vi "TEG P116x2w_Write_Manual.vi"(7 "MaxOutput":T1={"Ch1"=100.0, "Ch2"=100.0}, 8 "error in (no error)":errorcluster, 9 "RateSP":T1, 10 "NuevoSP":T1, 11 "Comunicaciones":T2={"Alicats"="ASRL6::INSTR", "Alic"=FALSE, "eValve"="ASRL6::INSTR", "eval"=FALSE, "Eurotherm"="ASRL6::INSTR", "euro"=FALSE, "Cell GAS"="ASRL6::INSTR", "cgas"=FALSE, "Cell H2S"="ASRL6::INSTR", "ch2s"=FALSE}) -> (0 "error out":errorcluster, 1 "RateSP(C/min) 2":T1, 2 "NuevoSP(C) 2":T1, 3 "MaxOutput 2":T1)   [LabVIEW 2017]
uses:
  2xP116.ctl
  REACTOR_COMUNICACIONES.ctl
  Eurotherm_2023_Module.ctl
  REACTOR_GLOBALES.vi
panel:
  out "Temp":T1
  in  "Cancel":bool
  in  "OK":bool
  out "Enable(T)":bool=TRUE
  out "VISA Promux":refnum<visa-resource-name>
  in  "Delay Time (s)":dbl=0.1
  # "Programando controladores P116"
  # "C"
  # "%"
  # "CALOR"
  # "C/min"
  # "C"
  # "%"
  # "FRIO"
  # "C/min"
  # "NOTA: La válvula de \"aire frio\" se conectará cuando \nla temperatura del reactor supere la temperatura \nNuevoSP FRIO establecida"
  # "Abril 2023 V1.0  a-sslcdms"
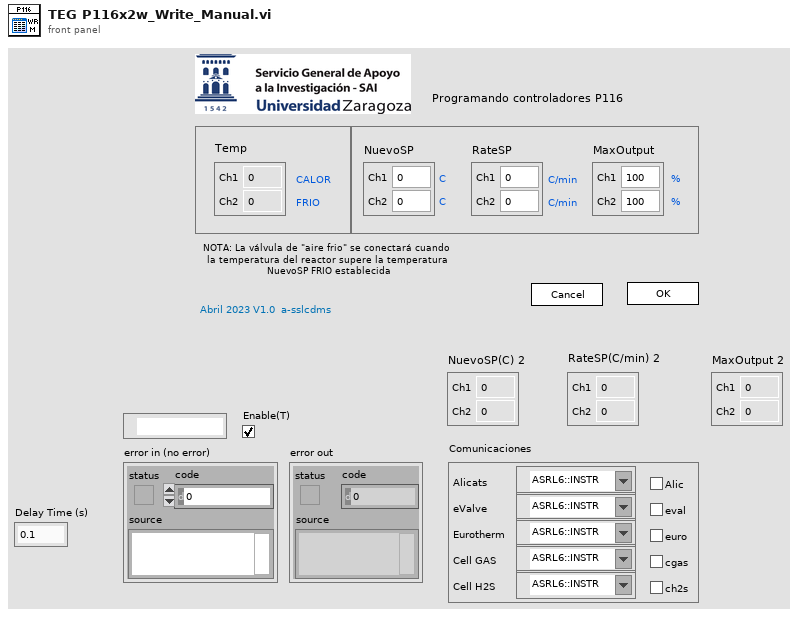
[diagram p1: front panel]
types:
  T1 = typedef "2xP116.ctl" = cluster{"Ch1":dbl, "Ch2":dbl}
  T2 = typedef "REACTOR_COMUNICACIONES.ctl" = cluster{"Alicats":refnum<visa-resource-name>, "Alic":bool, "eValve":refnum<visa-resource-name>, "eval":bool, "Eurotherm":refnum<visa-resource-name>, "euro":bool, "Cell GAS":refnum<visa-resource-name>, "cgas":bool, "Cell H2S":refnum<visa-resource-name>, "ch2s":bool}
  T3 = typedef "TEG P116x2w.ctl" = cluster{"TargetSP":T1, "WorkingSP":T1, "Temperatura":T1, "Error":bool, "Date":string, "Delay(s)":dbl, "RateSP":T1, "Potencia":T1, "Potencia max":T1}
  T4 = typedef "Eurotherm_2023_Module.ctl" = enum16{"Initialize", "Write setpoint", "Read data", "Write ramp rate", "Set constante proporcional", "Set constante integral", "Set constante diferencial", "Set ouput limit LOW", "Set ouput limit HIGH", "Shutdown"}
  T5 = enum16{"Add 1", "Add 2", "Add 3", "Add 10", "Add 11", "Add 12", "Add 13"}[]
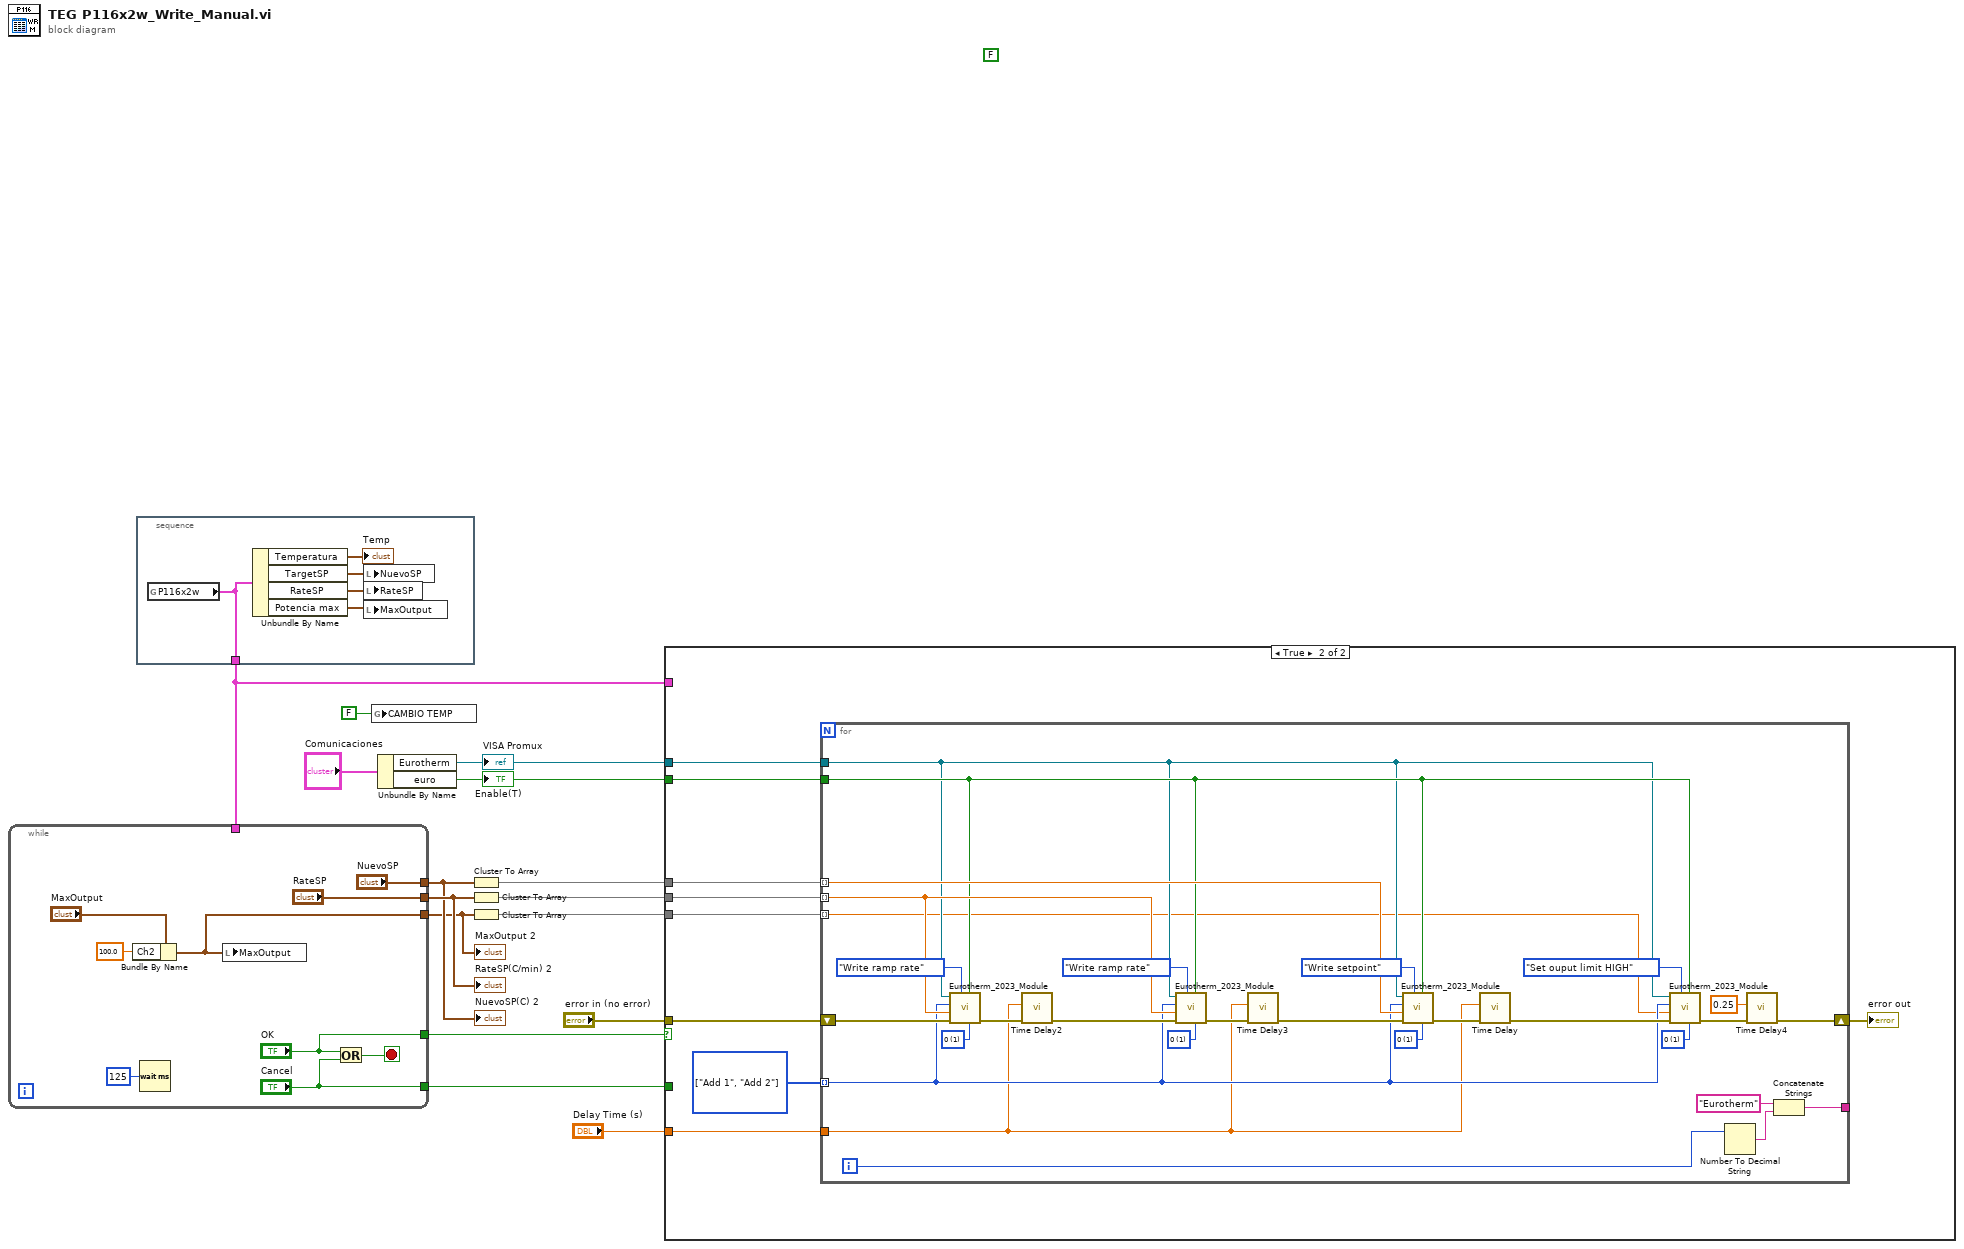
[diagram p0: block diagram]
diagram:
  (unwired) FALSE
  n1 = stacked-sequence {
    tunnel: [w18] -> w7
    frame #0 {
      n2 = global read "REACTOR_GLOBALES.vi" "P116x2w"() -> (w18:T3)
      n3 = Unbundle By Name(w18) -> ("Temperatura"=→"Temp":T1, "TargetSP"=w19:T1, "RateSP"=w17:T1, "Potencia max"=w16:T1)
      n4 = local write "NuevoSP"(w19) -> ()
      n5 = local write "RateSP"(w17) -> ()
      n6 = local write "MaxOutput"(w16) -> ()
    }
  }
  n7 = while {
    tunnel: ["Cancel"] -> w14
    tunnel: ["NuevoSP"] -> w3
    tunnel: ["RateSP"] -> w6
    tunnel: ["OK"] -> w10
    tunnel: w7 -> [_]
    tunnel: [w21] -> w2
    stop <- w24 stop-if-true
    n8 = Bundle By Name(cluster="MaxOutput", "Ch2"=100.0) -> (w21:T1)
    n9 = Wait (ms)(milliseconds to wait=u32 125) -> ()  [unwired: 1 out]
    n10 = local write "MaxOutput"(w21) -> ()
    n11 = Or(x="OK", y="Cancel") -> (x .or. y?=w24:bool)
  }
  "NuevoSP(C) 2" <- w3
  "RateSP(C/min) 2" <- w6
  "MaxOutput 2" <- w2
  n12 = global write "REACTOR_GLOBALES.vi" "CAMBIO TEMP"(FALSE ("ChangeT")) -> ()
  n13 = Unbundle By Name("Comunicaciones") -> ("Eurotherm"=w8:refnum<visa-resource-name>, "euro"=w15:bool)
  "Enable(T)" <- w15
  "VISA Promux" <- w8
  n14 = Cluster To Array(cluster=w3) -> (array=w12:dbl[])
  n15 = Cluster To Array(cluster=w6) -> (array=w11:dbl[])
  n16 = Cluster To Array(cluster=w2) -> (array=w4:dbl[])
  n17 = case shown="True" w10 {
    tunnel: w15 -> [_ w37]
    tunnel: w14 -> [_ _]
    tunnel: "error in (no error)" -> [_ w35]
    tunnel: w12 -> [_ w33]
    tunnel: w11 -> [_ w34]
    tunnel: w8 -> [_ w38]
    tunnel: w7 -> [_ _]
    tunnel: w4 -> [_ w31]
    tunnel: "Delay Time (s)" -> [_ w30]
    frame False {
    }
    frame True {
      w32 = T5 [enum."Add 1", enum."Add 2"] items=["Add 1", "Add 2", "Add 3", "Add 10", "Add 11", "Add 12", "Add 13"]
      n18 = for {
        shift-right: [w45] -> w36
        shift-left: w35 -> [w62]
        tunnel: [w65] -> _
        tunnel: w33 -> [w61] mode=indexing
        tunnel: w34 -> [w50] mode=indexing
        tunnel: w38 -> [w43]
        tunnel: w37 -> [w44]
        tunnel: w32 -> [w42] mode=indexing
        tunnel: w31 -> [w39] mode=indexing
        tunnel: w30 -> [w41]
        i -> [w59]
        w49 = u16 1 items=["0"=1, "1"=10, "2"=100] ("Decimales")
        w54 = u16 1 items=["0"=1, "1"=10, "2"=100] ("Decimales")
        w58 = u16 1 items=["0"=1, "1"=10, "2"=100] ("Decimales")
        w57 = u16 1 items=["0"=1, "1"=10, "2"=100] ("Decimales")
        n19 = call "Eurotherm_2023_Module.vi"("Decimales"=w58, "Eurotherm (T:Enable)"=w44, "Command"=Eurotherm_2023_Module."Write ramp rate", "error in (no error)"=w62, "Value"=w50, "Address"=w42, "VISA resource name"=w43) -> ("error out"=w56:errorcluster)  [unwired: 3 in, 1 out]
        n20 = call "Time Delay2"("error in (no error)"=w56, "Delay Time (s)"=w41) -> ("error out"=w52:errorcluster)  [unwired: 9 in]
        n21 = call "Eurotherm_2023_Module.vi"("Decimales"=w54, "Eurotherm (T:Enable)"=w44, "Command"=Eurotherm_2023_Module."Write ramp rate", "error in (no error)"=w52, "Value"=w50, "Address"=w42, "VISA resource name"=w43) -> ("error out"=w55:errorcluster)  [unwired: 3 in, 1 out]
        n22 = call "Time Delay3"("error in (no error)"=w55, "Delay Time (s)"=w41) -> ("error out"=w51:errorcluster)  [unwired: 9 in]
        n23 = call "Eurotherm_2023_Module.vi"("Decimales"=w57, "Eurotherm (T:Enable)"=w44, "Command"=Eurotherm_2023_Module."Write setpoint", "error in (no error)"=w51, "Value"=w61, "Address"=w42, "VISA resource name"=w43) -> ("error out"=w60:errorcluster)  [unwired: 3 in, 1 out]
        n24 = call "Time Delay"("error in (no error)"=w60, "Delay Time (s)"=w41) -> ("error out"=w46:errorcluster)  [unwired: 9 in]
        n25 = call "Eurotherm_2023_Module.vi"("Decimales"=w49, "Eurotherm (T:Enable)"=w44, "Command"=Eurotherm_2023_Module."Set ouput limit HIGH", "error in (no error)"=w46, "Value"=w39, "Address"=w42, "VISA resource name"=w43) -> ("error out"=w48:errorcluster)  [unwired: 3 in, 1 out]
        n26 = Number To Decimal String(number=w59) -> (decimal integer string=w66:string)  [unwired: 1 in]
        n27 = call "Time Delay4"("error in (no error)"=w48, "Delay Time (s)"=0.25) -> ("error out"=w45:errorcluster)  [unwired: 9 in]
        n28 = Concatenate Strings("Eurotherm" ("error source (\" \")"), w66) -> (w65:string)
      }
      "error out" <- w36
    }
  }
